vi "Variant To Control__A2E.vi"(7 "Control VI Type (control)":T1=enum."control" caption="Control VI Type", 8 "Error In":errorcluster, 10 "Variant Data":variant, 11 "Control Path (use dialog)":path) -> (0 "error out":errorcluster, 3 "selected path":path)   [LabVIEW 2021, in "Utilities.lvlib"]
doc: "Converts any datatype into a control.\nThis control can be a (strict) TypeDef"
uses:
  Utilities.lvlib
  ControlTypes__A2E.ctl
  Instance           1 31Saved   Variant To Control__A2E .vi
  Instance           2 31Saved   Variant To Control__A2E .vi
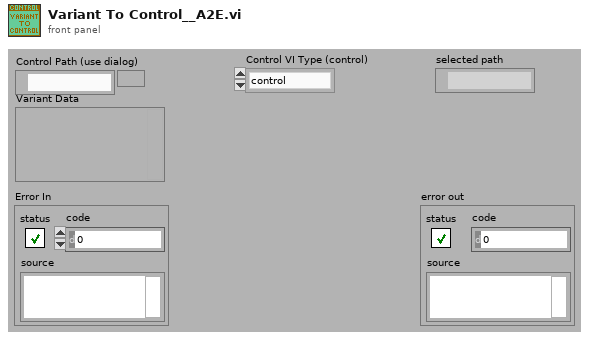
[diagram p1: front panel]
types:
  T1 = typedef "Utilities.lvlib/ControlTypes__A2E.ctl" = enum32{"not a control VI", "control", "typedef", "strict typedef"}
  T2 = enum32{"invalid VI type", "Standard VI", "Control VI", "Global VI", "Polymorphic VI"}
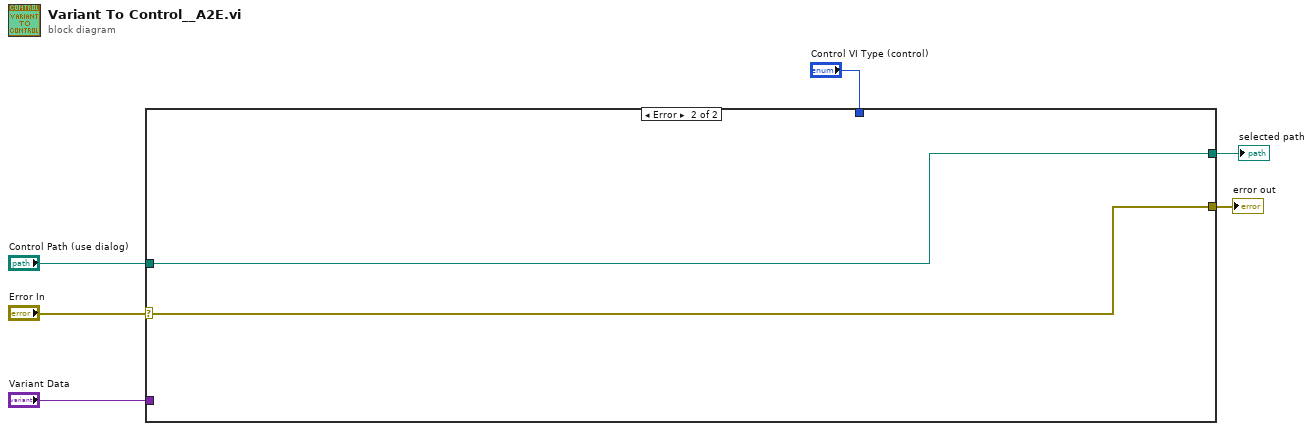
[diagram p0: block diagram]
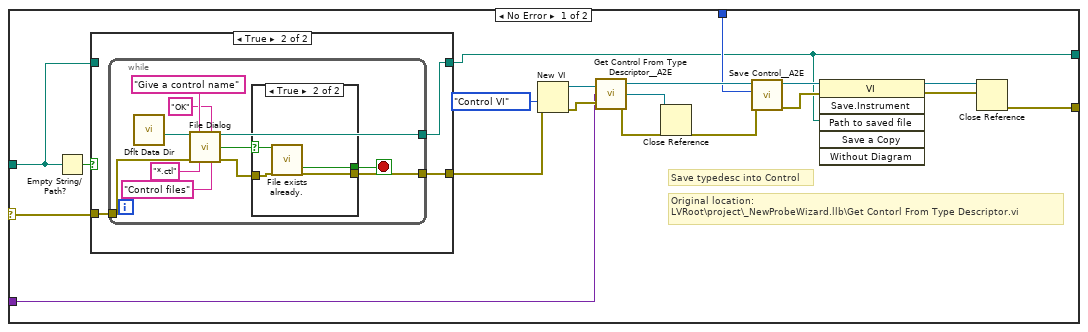
[diagram p2: hidden frame]
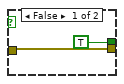
[diagram p4: hidden frame]
diagram:
  n1 = case shown="Error" "Error In" {
    selector: "Error In" -> [w7 w48]
    tunnel: "Control Path (use dialog)" -> [w25 w49]
    tunnel: "Variant Data" -> [w16 _]
    tunnel: "Control VI Type (control)" -> [w14 _]
    tunnel: [w10 w48] -> w3
    tunnel: [w9 w49] -> w2
    frame No Error {
      # "Original location:\nLVRoot\\project\\_NewProbeWizard.llb\\Get Contorl From Type Descriptor.vi"
      # "Save typedesc into Control"
      n2 = Empty String/Path?(string/path=w25) -> (empty?=w8:bool)
      n3 = case shown="True" w8 {
        tunnel: w7 -> [w27 w30]
        tunnel: [w27 w29] -> w15
        tunnel: [w26 w28] -> w9
        tunnel: w25 -> [w26 _]
        frame False {
        }
        frame True {
          n4 = while {
            tunnel: w30 -> [w37]
            tunnel: [w32] -> w29
            tunnel: [w31] -> w28
            stop <- w33 stop-if-true
            n5 = call <vilib>:"Dflt Data Dir.vi"() -> ("App:Default Data Directory"=w36:path)
            n6 = call "File Dialog"("start path"=w36, "prompt"="Give a control name", "button label"="OK", "error in"=w37, "pattern (all files)"="*.ctl", "pattern label"="Control files") -> ("selected path"=w31:path, "exists"=w35:bool, "error out"=w34:errorcluster)  [unwired: 6 in, 1 out]
            n7 = case shown="True" w35 {
              selector: w35 -> [_ w47]
              tunnel: w34 -> [w42 w46]
              tunnel: [TRUE ("Yes") w45] -> w33
              tunnel: [w42 w44] -> w32
              frame False {
              }
              frame True {
                n8 = call "File exists already."("Enable"=w47, "error in (no error)"=w46) -> ("Yes"=w45:bool, "error out"=w44:errorcluster)  [unwired: 16 in]
              }
            }
          }
        }
      }
      n9 = New VI(8:w15, 9:T2."Control VI" ("vi type (standard vi)")) -> (0:w24:errorcluster, 3:w17:refnum<vi>)  [unwired: 5 in]
      n10 = call "Get Control From Type Descriptor__A2E.vi"("VI Refnum"=w17, "error in (no error)"=w24, "data type"=w16) -> ("VI Refnum"=w18:refnum<vi>, "New Control Ref"=w20:refnum<vi>, "error out"=w19:errorcluster)
      n11 = Close Reference(reference=w20, error in (no error)=w19) -> (error out=w21:errorcluster)
      n12 = call "Save Control__A2E.vi"("error in (no error)"=w21, "Control VI Type"=w14, "vi reference in"=w18) -> ("error out"=w13:errorcluster, "vi reference out"=w12:refnum<vi>)  [unwired: 7 in]
      n13 = invoke class="VI" method="Save.Instrument"(reference=w12, error in=w13, "Path to saved file"=w9) -> (reference out=w22:refnum<vi>, error out=w23:errorcluster)  [unwired: 3 in, 4 out]
      n14 = Close Reference(reference=w22, error in (no error)=w23) -> (error out=w10:errorcluster)
    }
    frame Error {
    }
  }
  "error out" <- w3
  "selected path" <- w2
